vi "CRYPreLoad StepRefs.vi"() -> (0 "End Flag?":bool=TRUE)   [LabVIEW 2013]
uses:
  CRYSystem/Program/CRYRef nums global.vi
  CRYMainGlobal.vi
  CRYWindow/SubVI/CRYMain Sub Window Global.vi
panel:
  in  "type specifier VI Refnum (for type only)":refnum<vi>
  in  "type specifier":refnum<vi>
  # "Load used *.vi front panel interface language setting."
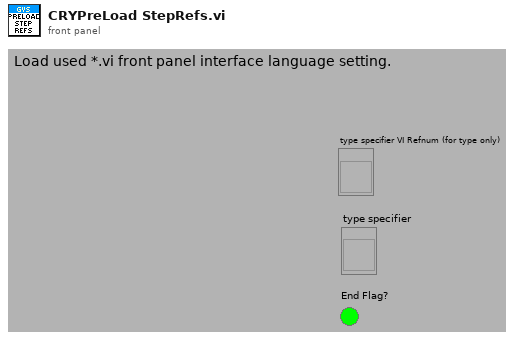
[diagram p1: front panel]
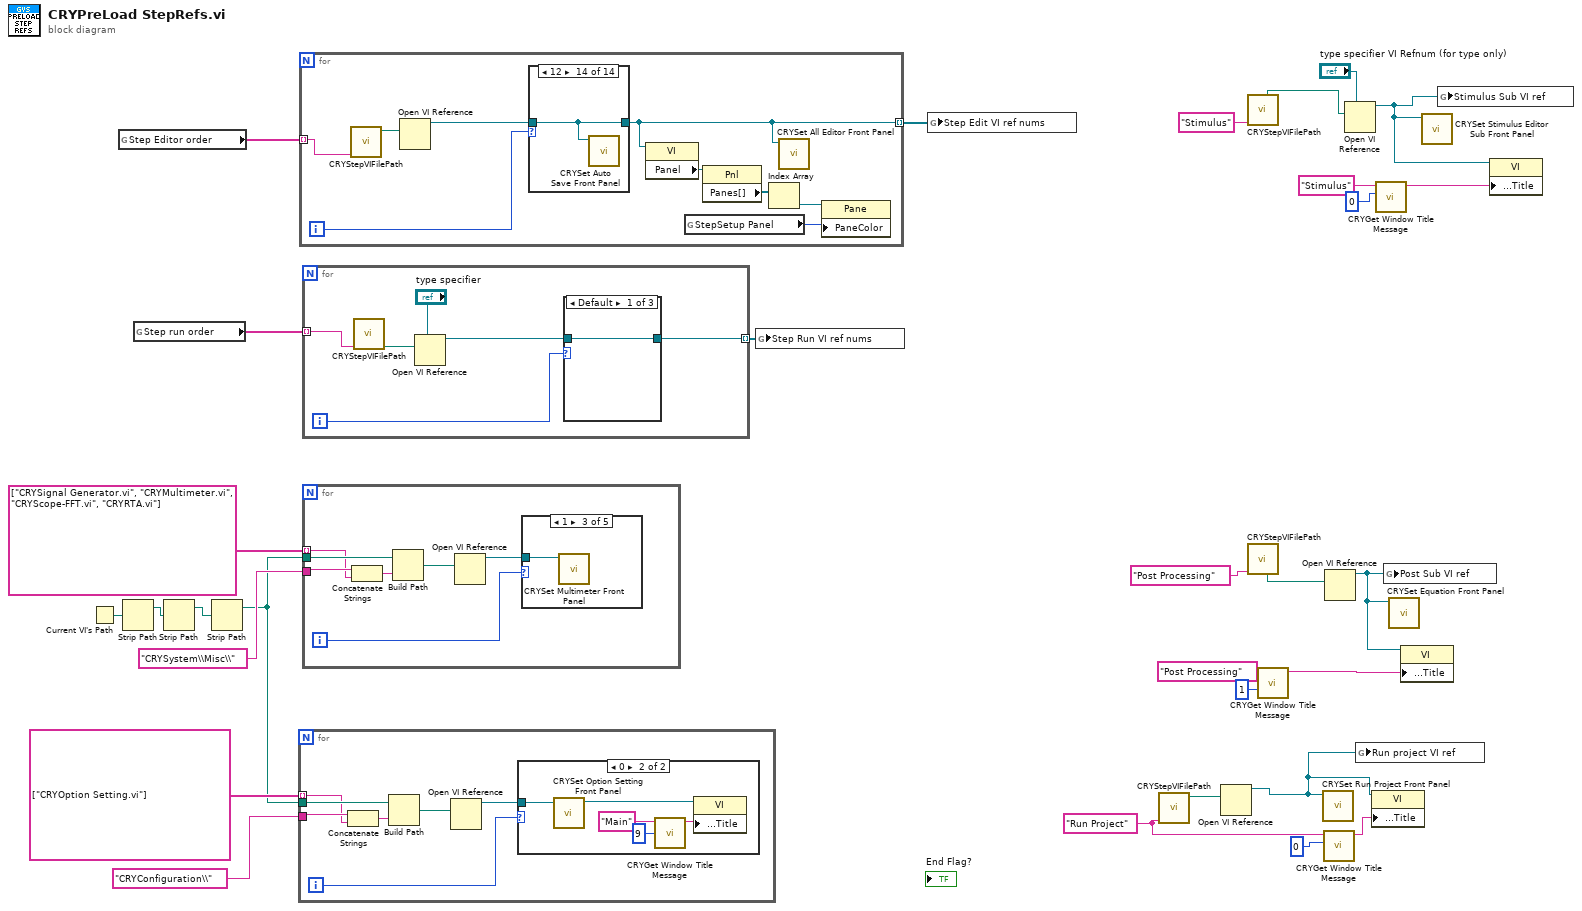
[diagram p0: block diagram]
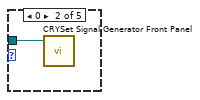
[diagram p3: hidden frame]
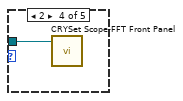
[diagram p4: hidden frame]
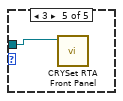
[diagram p5: hidden frame]
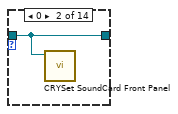
[diagram p8: hidden frame]
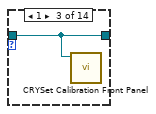
[diagram p9: hidden frame]
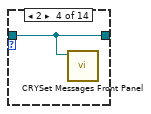
[diagram p10: hidden frame]
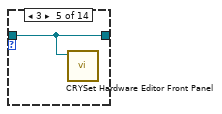
[diagram p11: hidden frame]
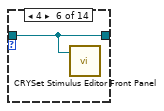
[diagram p12: hidden frame]
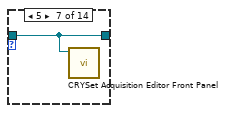
[diagram p13: hidden frame]
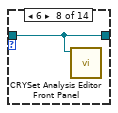
[diagram p14: hidden frame]
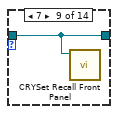
[diagram p15: hidden frame]
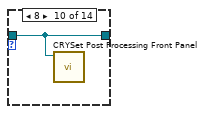
[diagram p16: hidden frame]
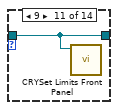
[diagram p17: hidden frame]
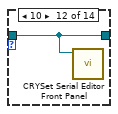
[diagram p18: hidden frame]
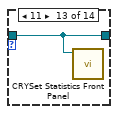
[diagram p19: hidden frame]
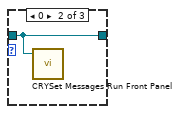
[diagram p20: hidden frame]
diagram:
  w27 = "Run Project" ("Name")
  n1 = Current VI's Path() -> (path=w7:path)
  n2 = global read "CRYMainGlobal.vi" "Step Editor order"() -> (w3:string[])
  n3 = Strip Path(path=w7) -> (stripped path=w6:path)  [unwired: 1 out]
  n4 = global read "CRYMainGlobal.vi" "Step run order"() -> (w10:string[])
  n5 = Strip Path(path=w6) -> (stripped path=w5:path)  [unwired: 1 out]
  n6 = Strip Path(path=w5) -> (stripped path=w4:path)  [unwired: 1 out]
  n7 = for {
    tunnel: string[] ["CRYOption Setting.vi"] ("Step run order") -> [w32] mode=indexing
    tunnel: w4 -> [w35]
    tunnel: "CRYConfiguration\\" -> [w33]
    i -> [w36]
    n8 = Concatenate Strings(w33, w32) -> (w31:string)
    n9 = Build Path(base path=w35, name or relative path=w31) -> (appended path=w34:path)
    n10 = Open VI Reference(vi path=w34) -> (vi reference=w37:refnum<vi>)  [unwired: 5 in, 1 out]
    n11 = case shown="0" w36 {
      tunnel: w37 -> [_ w42]
      frame Default {
      }
      frame 0 {
        n12 = call "CRYSet Option Setting Front Panel.vi"("Vi Ref in"=w42) -> ("Vi Ref out"=w38:refnum<vi>)  [unwired: 10 in]
        n13 = call "CRYGet Window Title Message.vi"("No"=9, "Kind"="Main") -> ("Multibyte String"=w39:string)  [unwired: 4 in, 5 out]
        n14 = property class="VI"(reference=w38, "Front Panel.Title"=w39) -> ()  [unwired: 1 in, 2 out]
      }
    }
  }
  n15 = for {
    tunnel: w3 -> [w51] mode=indexing
    tunnel: [w43] -> w25 mode=indexing
    i -> [w50]
    n16 = call "CRYStepVIFilePath.vi"("Category Name"=w51) -> ("Editor VI Path Out"=w48:path)  [unwired: 1 in, 8 out]
    n17 = Open VI Reference(vi path=w48) -> (vi reference=w49:refnum<vi>)  [unwired: 5 in, 1 out]
    n18 = case shown="12" w50 {
      tunnel: w49 -> [w52 w53 w54 w55 w56 w57 w58 w59 w60 w61 w62 w63 w64 w65]
      tunnel: [w52 w53 w54 w55 w56 w57 w58 w59 w60 w61 w62 w63 w64 w65] -> w43
      frame Default {
      }
      frame 0 {
        n19 = call "CRYSet SoundCard Front Panel.vi"("Vi Ref in"=w53) -> ()  [unwired: 10 in, 1 out]
      }
      frame 1 {
        n20 = call "CRYSet Calibration Front Panel.vi"("Vi Ref"=w54) -> ()  [unwired: 11 in]
      }
      frame 2 {
        n21 = call "CRYSet Messages Front Panel.vi"("Vi Ref"=w55) -> ()  [unwired: 11 in]
      }
      frame 3 {
        n22 = call "CRYSet Hardware Editor Front Panel.vi"("Vi Ref"=w56) -> ()  [unwired: 11 in]
      }
      frame 4 {
        n23 = call "CRYSet Stimulus Editor Front Panel.vi"("Vi Ref"=w57) -> ()  [unwired: 11 in]
      }
      frame 5 {
        n24 = call "CRYSet Acquisition Editor Front Panel.vi"("Vi Ref"=w58) -> ()  [unwired: 11 in]
      }
      frame 6 {
        n25 = call "CRYSet Analysis Editor Front Panel.vi"("Vi Ref"=w59) -> ()  [unwired: 11 in]
      }
      frame 7 {
        n26 = call "CRYSet Recall Front Panel.vi"("Vi Ref"=w60) -> ()  [unwired: 11 in]
      }
      frame 8 {
        n27 = call "CRYSet Post Processing Front Panel.vi"("Vi Ref"=w61) -> ()  [unwired: 11 in]
      }
      frame 9 {
        n28 = call "CRYSet Limits Front Panel.vi"("Vi Ref"=w62) -> ()  [unwired: 11 in]
      }
      frame 10 {
        n29 = call "CRYSet Serial Editor Front Panel.vi"("Vi Ref"=w63) -> ()  [unwired: 11 in]
      }
      frame 11 {
        n30 = call "CRYSet Statistics Front Panel.vi"("Vi Ref"=w64) -> ()  [unwired: 11 in]
      }
      frame 12 {
        n31 = call "CRYSet Auto Save Front Panel.vi"("Vi Ref"=w65) -> ()  [unwired: 11 in]
      }
    }
    n32 = property on="Property Node" class="VI"(reference=w43) -> ("Panel"=w47:refnum<vi>)  [unwired: 1 in, 2 out]
    n33 = global read "CRYMain Sub Window Global.vi" "StepSetup Panel"() -> (w44:u32)
    n34 = property on="Property Node" class="Pnl"(reference=w47) -> ("Panes[]"=w46:refnum<vi>[])  [unwired: 1 in, 2 out]
    n35 = Index Array(array=w46) -> (element=w45:refnum<vi>)  [unwired: 1 in]
    n36 = call "CRYSet All Editor Front Panel.vi"("VI Ref"=w43) -> ()  [unwired: 11 in]
    n37 = property class="Pane"(reference=w45, "PaneColor"=w44) -> ()  [unwired: 1 in, 2 out]
  }
  n38 = for {
    tunnel: w10 -> [w71] mode=indexing
    tunnel: [w67] -> w2 mode=indexing
    i -> [w68]
    n39 = call "CRYStepVIFilePath.vi"("Category Name"=w71) -> ("Run VI Path Out"=w69:path)  [unwired: 1 in, 8 out]
    n40 = Open VI Reference(type specifier VI Refnum (for type only)="type specifier", vi path=w69) -> (vi reference=w66:refnum<vi>)  [unwired: 4 in, 1 out]
    n41 = case shown="Default" w68 {
      tunnel: w66 -> [w72 w73 w74]
      tunnel: [w72 w73 w74] -> w67
      frame Default {
      }
      frame 0 {
        n42 = call "CRYSet Messages Run Front Panel.vi"("Vi Ref"=w73) -> ()  [unwired: 11 in]
      }
      frame 7 {
        n43 = call "CRYSet Limits Run Front Panel.vi"("Vi Ref"=w74) -> ()  [unwired: 11 in]
      }
    }
  }
  n44 = for {
    tunnel: string[] ["CRYSignal Generator.vi", "CRYMultimeter.vi", "CRYScope-FFT.vi", "CRYRTA.vi"] ("Step run order") -> [w77] mode=indexing
    tunnel: w4 -> [w79]
    tunnel: "CRYSystem\\Misc\\" -> [w78]
    i -> [w80]
    n45 = Concatenate Strings(w78, w77) -> (w76:string)
    n46 = Build Path(base path=w79, name or relative path=w76) -> (appended path=w75:path)
    n47 = Open VI Reference(vi path=w75) -> (vi reference=w81:refnum<vi>)  [unwired: 5 in, 1 out]
    n48 = case shown="1" w80 {
      tunnel: w81 -> [_ w82 w83 w84 w85]
      frame Default {
      }
      frame 0 {
        n49 = call "CRYSet Signal Generator Front Panel.vi"("Vi Ref in"=w82) -> ()  [unwired: 10 in, 1 out]
      }
      frame 1 {
        n50 = call "CRYSet Multimeter Front Panel.vi"("Vi Ref in"=w83) -> ()  [unwired: 10 in, 1 out]
      }
      frame 2 {
        n51 = call "CRYSet Scope-FFT Front Panel.vi"("Vi Ref in"=w84) -> ()  [unwired: 10 in, 1 out]
      }
      frame 3 {
        n52 = call "CRYSet RTA Front Panel.vi"("Vi Ref in"=w85) -> ()  [unwired: 10 in, 1 out]
      }
    }
  }
  n53 = global write "CRYRef nums global.vi" "Step Run VI ref nums"(w2) -> ()
  n54 = global write "CRYRef nums global.vi" "Step Edit VI ref nums"(w25) -> ()
  n55 = call "CRYStepVIFilePath.vi"("Category Name"=w27) -> ("Editor VI Path Out"=w28:path)  [unwired: 1 in, 8 out]
  n56 = Open VI Reference(vi path=w28) -> (vi reference=w26:refnum<vi>)  [unwired: 1 in, 5 out]
  n57 = call "CRYStepVIFilePath.vi"("Category Name"="Stimulus" ("Content")) -> ("Special path"=w23:path)  [unwired: 1 in, 8 out]
  n58 = call "CRYStepVIFilePath.vi"("Category Name"="Post Processing" ("Content")) -> ("Special path"=w17:path)  [unwired: 1 in, 8 out]
  n59 = call "CRYGet Window Title Message.vi"("No"=1, "Kind"="Post Processing") -> ("Multibyte String"=w14:string)  [unwired: 4 in, 5 out]
  n60 = call "CRYSet Run Project Front Panel.vi"("Vi Ref in"=w26) -> ()  [unwired: 10 in, 1 out]
  n61 = call "CRYGet Window Title Message.vi"("No"=0 ("Error No"), "Kind"=w27) -> ("Multibyte String"=w30:string)  [unwired: 4 in, 5 out]
  n62 = Open VI Reference(vi path=w17) -> (vi reference=w13:refnum<vi>)  [unwired: 1 in, 5 out]
  n63 = Open VI Reference(type specifier VI Refnum (for type only)="type specifier VI Refnum (for type only)", vi path=w23) -> (vi reference=w1:refnum<vi>)  [unwired: 4 in, 1 out]
  n64 = global write "CRYRef nums global.vi" "Run project VI ref"(w26) -> ()
  n65 = property class="VI"(reference=w26, "Front Panel.Title"=w30) -> ()  [unwired: 1 in, 2 out]
  n66 = call "CRYGet Window Title Message.vi"("No"=0, "Kind"="Stimulus" ("Front Panel Window:Title")) -> ("Multibyte String"=w20:string)  [unwired: 4 in, 5 out]
  n67 = global write "CRYRef nums global.vi" "Post Sub VI ref"(w13) -> ()
  n68 = call "CRYSet Equation Front Panel.vi"("Vi Ref"=w13) -> ()  [unwired: 11 in]
  n69 = property class="VI"(reference=w13, "Front Panel.Title"=w14) -> ()  [unwired: 1 in, 2 out]
  n70 = call "CRYSet Stimulus Editor Sub Front Panel.vi"("Vi Ref"=w1) -> ()  [unwired: 11 in]
  n71 = global write "CRYRef nums global.vi" "Stimulus Sub VI ref"(w1) -> ()
  n72 = property class="VI"(reference=w1, "Front Panel.Title"=w20) -> ()  [unwired: 1 in, 2 out]
